vi "Stop.vi"(8 "error in (no error)":errorcluster, 10 "Message in":refnum<class "StopMessage.lvclass">, 11 "Tomo in":refnum<class "Tomo.lvclass">) -> (0 "error out":errorcluster, 3 "Tomo out":refnum<class "Tomo.lvclass">)   [LabVIEW 2012, in "Tomo.lvclass"]
doc: "This member function is called when the statemachine in the run.vi receives an 'stop' command. It relays the message to all observers of the component.\n\nOverride this member function in your derived class if you need additional stop functionality (but don't forget to call the parent method)."
uses:
  Tomo.lvclass
  <vilib>/Distrio/Murmex/StopMessage/StopMessage.lvclass
  Current activity.ctl
  Tomo.lvclass/Tomo.ctl
  notice type.ctl
  <vilib>/Distrio/Murmex/Murmex/Murmex.lvclass
panel:
  # "This method is called when the STOP\ntrigger is sent. \n\nOverride this method when your component needs to\nrespond to this trigger. \n\nCall parent for proper implementation"
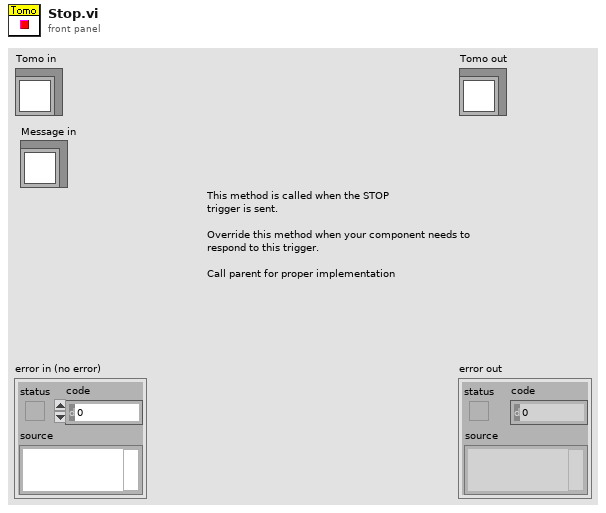
[diagram p1: front panel]
types:
  T1 = typedef "Tomo.lvclass/Current activity.ctl" = enum16{"Idle", "Inter-stack motion", "Autofocus", "Stack acquisition"}
  T2 = typedef "Tomo.lvclass/notice type.ctl" = enum16{"Tomography stopped", "Tomography error", "Tomography finished", "Timing issue", "Critical timing issue"}
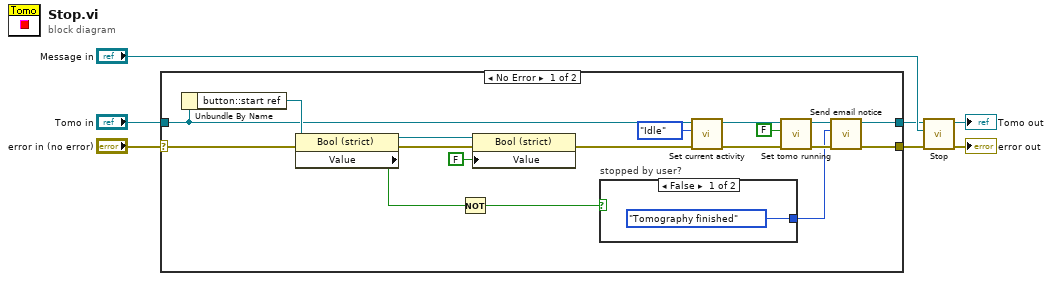
[diagram p0: block diagram]
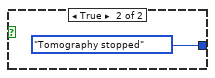
[diagram p2: hidden frame]
diagram:
  n1 = case shown="No Error" "error in (no error)" {
    selector: "error in (no error)" -> [w25 w29]
    tunnel: [w18 w29] -> w3
    tunnel: "Tomo in" -> [w10 w28]
    tunnel: [w16 w28] -> w1
    frame No Error {
      n2 = Unbundle By Name(w10) -> ("button::start ref"=w20:refnum<vi>)
      n3 = property class="Bool (strict)"(reference=w20, error in=w25) -> (reference out=w19:refnum<vi>, error out=w21:errorcluster, "Value"=w15:bool)
      n4 = Not(x=w15) -> (.not. x?=w13:bool)
      n5 = property class="Bool (strict)"(reference=w19, error in=w21, "Value"=FALSE) -> (error out=w9:errorcluster)  [unwired: 1 out]
      n6 = case "stopped by user?" shown="False" w13 {
        tunnel: [notice_type."Tomography finished" ("Notice type") notice_type."Tomography stopped" ("Notice type")] -> w14
        frame False {
        }
        frame True {
        }
      }
      n7 = call-dynamic "Set current activity.vi"("error in (no error)"=w9, "Current activity"=Current_activity."Idle", "Tomo in"=w10) -> ("error out"=w12:errorcluster, "Tomo out"=w11:refnum<class "Tomo.lvclass">)  [unwired: 7 in]
      n8 = call-dynamic "Set tomo running.vi"("error in (no error)"=w12, "tomo running?"=FALSE, "Tomo in"=w11) -> ("error out"=w23:errorcluster, "Tomo out"=w17:refnum<class "Tomo.lvclass">)  [unwired: 7 in]
      n9 = call-dynamic "Send email notice.vi"("error in (no error)"=w23, "Notice type"=w14, "Tomo in"=w17) -> ("error out"=w18:errorcluster, "Tomo out"=w16:refnum<class "Tomo.lvclass">)  [unwired: 7 in]
    }
    frame Error {
    }
  }
  n10 = call-parent "Stop.vi"("error in (no error)"=w3, "Message in"="Message in", "Murmex in"=w1) -> ("error out"=→"error out":errorcluster, "Murmex out"=→"Tomo out":refnum<class "Tomo.lvclass">)  [unwired: 7 in]
